vi "MultiGaussModel.vi"(3 "output control":T1, 4 "data":T2, 5 "X":dbl[](array[numeric]), 6 "a":dbl[](array[numeric])) -> (0 "error out":errorcluster, 1 "f'(X,a)":dbl[][](array[numeric]), 2 "f(X,a)":dbl[](array[numeric]))   [LabVIEW 2015]
doc: "This template is the starting point for creating a model function to be passed to the Nonlinear Curve Fit.vi."
uses:
  <vilib>/gmath/NumericalOptimization/objective function data.ctl
  <vilib>/gmath/NumericalOptimization/LM_output select.ctl
  <vilib>/gmath/NI_Gmath.lvlib
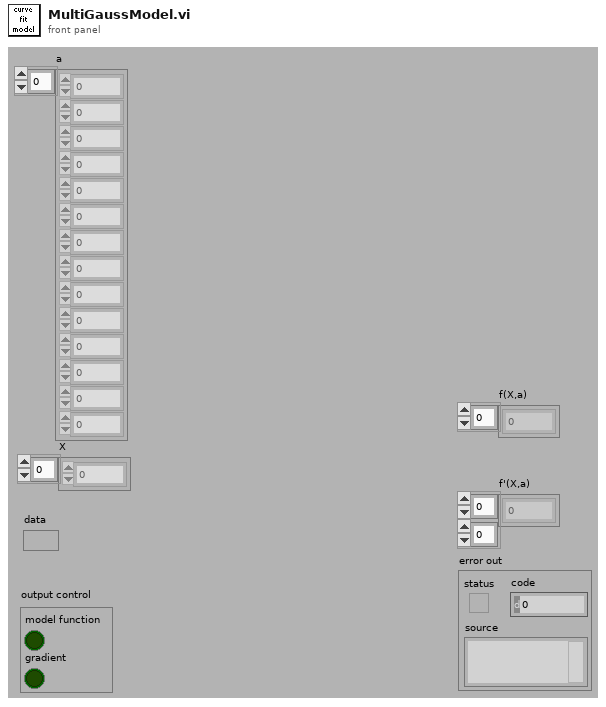
[diagram p1: front panel]
types:
  T1 = typedef "NI_Gmath.lvlib/LM_output select.ctl" = cluster{"model function":bool, "gradient":bool}
  T2 = typedef "NI_Gmath.lvlib/objective function data.ctl" = variant
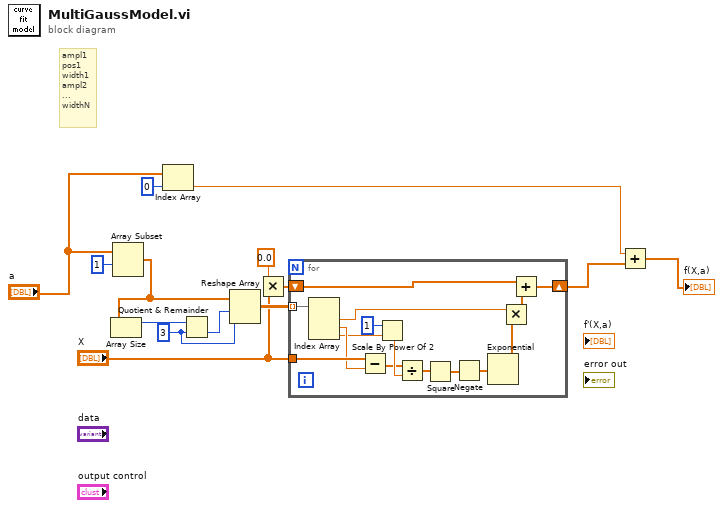
[diagram p0: block diagram]
diagram:
  w14 = 3 ("y")
  # "ampl1\npos1\nwidth1\nampl2\n...\nwidthN"
  n1 = Array Subset(array="a", index=1) -> (w4:dbl[])  [unwired: 1 in]
  n2 = Array Size(array=w4) -> (size(s)=w5:i32)
  n3 = Index Array(array="a", index=0) -> (element=w3:dbl)
  n4 = Quotient & Remainder(x=w5, y=w14) -> (floor(x/y)=w13:i32)  [unwired: 1 out]
  n5 = Reshape Array(w4, w13, w14) -> (w12:dbl[][])
  n6 = Multiply(x=0.0, y="X") -> (x*y=w9:dbl[])
  n7 = for {
    tunnel: "X" -> [w28]
    tunnel: w12 -> [w25] mode=indexing
    shift-right: [w18] -> w2
    shift-left: w9 -> [w19]
    n8 = Index Array(array=w25) -> (element #1=w22:dbl, element #2=w24:dbl, element #3=w23:dbl)  [unwired: 3 in]
    n9 = Subtract(x=w28, y=w24) -> (x-y=w17:dbl[])
    n10 = Scale By Power Of 2(n=i16 1, x=w23) -> (x*2^n=w27:dbl)
    n11 = Divide(x=w17, y=w27) -> (x/y=w26:dbl[])
    n12 = Square(x=w26) -> (x^2=w16:dbl[])
    n13 = Negate(x=w16) -> (-x=w15:dbl[])
    n14 = Exponential(1:w15) -> (0:w21:dbl[])
    n15 = Multiply(x=w22, y=w21) -> (x*y=w20:dbl[])
    n16 = Add(x=w19, y=w20) -> (x+y=w18:dbl[])
  }
  n17 = Add(x=w3, y=w2) -> (x+y=→"f(X,a)":dbl[])
